vi "softmax.vi"(1 "Array":dbl[](array[numeric])) -> (0 "softmax":dbl[](array[numeric]))   [LabVIEW 2023]
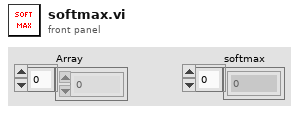
[diagram p1: front panel]
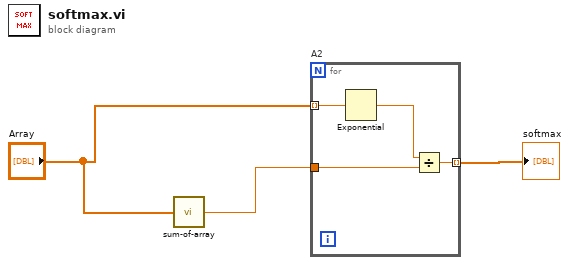
[diagram p0: block diagram]
diagram:
  n1 = call "sum-of-array.vi"("Array"="Array") -> ("sum of array"=w1:dbl)
  n2 = for "A2" {
    tunnel: "Array" -> [w7] mode=indexing
    tunnel: [w5] -> w3 mode=indexing
    tunnel: w1 -> [w4]
    n3 = Exponential(1:w7) -> (0:w6:dbl)
    n4 = Divide(x=w6, y=w4) -> (x/y=w5:dbl)
  }
  "softmax" <- w3
